vi "Periodic Tasks.vi"(8 "error in":errorcluster) -> ()   [LabVIEW 2013]
doc: "This VI runs in parallel to other tasks. It can contain as many user-defined periodic loops as you need. These can carry out PID or other sorts of timed response."
uses:
  <vilib>/Rock Robotics/SystemInterfaces/Typedef/FPGA_TypedefAnalogModule.ctl
  <vilib>/Rock Robotics/SystemInterfaces/Utilities/FPGA_UtilitiesLED Source.ctl
  <vilib>/Rock Robotics/SystemInterfaces/Utilities/FPGA_UtilitiesLED State.ctl
  <vilib>/Rock Robotics/WPI/Compressor/WPI_CompressorGetSetRefNum.vi
  Robot Global Data.vi
  <vilib>/Rock Robotics/WPI/RobotDrive/WPI_RobotDriveGetSetRefNum.vi
  <vilib>/Rock Robotics/WPI/Joystick/WPI_JoystickGetSetRefNum.vi
panel:
  out "distance":dbl(slide)=125.0 scale=0.0..250.0 scale format="%3d"
  in  "Scaling factor (V/in)":dbl=0.0098
  in  "Samples Per Second":dbl=1000.0
  in  "Average Bits":u8=3 max=15
  out "Encoder Rate (distance/sec)":dbl
  out "Encoder Distance":dbl
  out "Encoder Alarm Status":string
  out "Encoder Direction":string
  in  "Reset Encoder?":bool
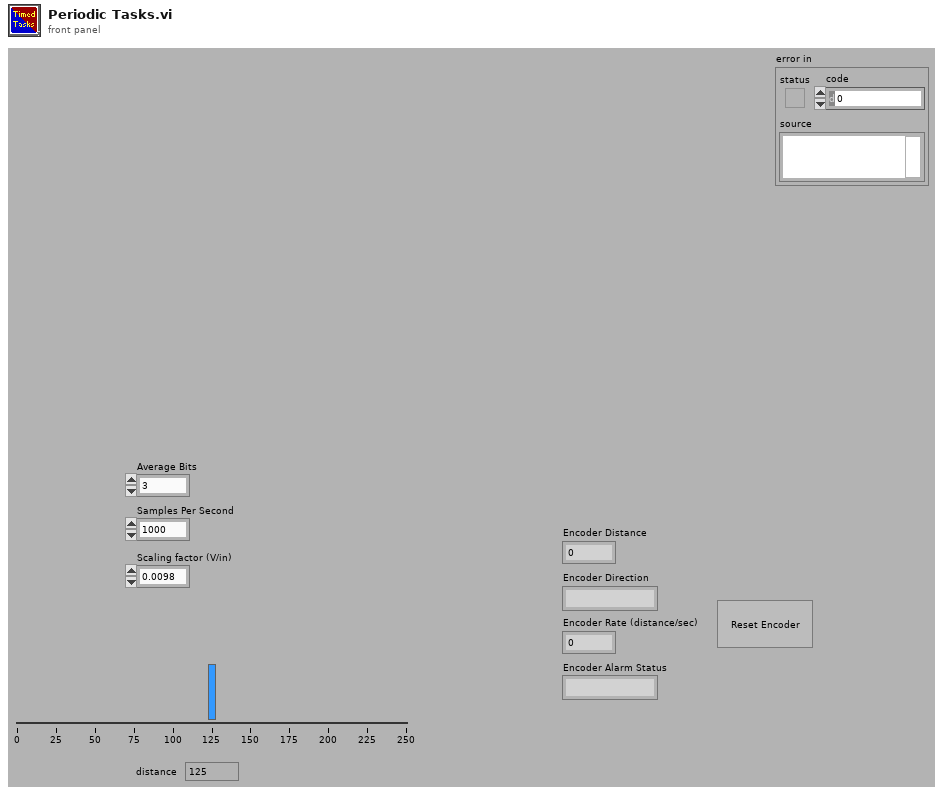
[diagram p1: front panel]
types:
  T1 = typedef "WPI_JoystickDevRef.ctl" = cluster{"Device":T2}
  T2 = typedef "WPI_JoystickDeviceEnum.ctl" = enum16{"USB 1", "USB 2", "USB 3", "USB 4", "Kinect 1", "Kinect 2"}
  T3 = typedef "WPI_RobotDriveDevRef.ctl" = cluster{"DevStatus":errorcluster, "Motors[]":T4[], "Square Inputs":bool, "Max Output":dbl, "Isochronous":bool}
  T4 = typedef "WPI_MotorControlDeviceRef.ctl" = cluster{"DeviceStatus":errorcluster, "Type":enum16{"PWM", "CAN"}, "PWM":cluster{"Digital Module":T5, "PWM Channel":T6, "DeadBand":T7}, "CAN":cluster{"Device Number":u8, "Control Mode":T8, "Semaphore":T9, "Max Vout":dbl}, "Invert":bool, "TransformRef":T10, "InvTransformRef":T10}
  T5 = typedef "FPGA_TypedefDigitalModule.ctl" = enum16{"Digital Module 1", "Digital Module 2"}
  T6 = typedef "FPGA_DIOPWMChannel.ctl" = enum8{"PWM 1", "PWM 2", "PWM 3", "PWM 4", "PWM 5", "PWM 6", "PWM 7", "PWM 8", "PWM 9", "PWM 10", "Invalid"}
  T7 = typedef "WPI_PWMDeadband.ctl" = cluster{"Name":string, "maxPositivePwm":i32, "minPositivePwm":i32, "centerPwm":i32, "maxNegativePwm":i32, "minNegativePwm":i32, "angularRange":u16}
  T8 = typedef "WPI_CANJaguar_ControlMode.ctl" = enum8{"Percent VBus", "Current", "Speed", "Position", "Voltage"}
  T9 = typedef "Semaphore RefNum" = refnum<k1>
  T10 = typedef "WPI_PWMTransform_ConPane.ctl" = refnum<vi>
  T11 = typedef "WPI_AnalogChannelDevRef.ctl" = cluster{"DevStatus":errorcluster, "Analog Module":T12, "Analog Channel":T13}
  T12 = typedef "FPGA_TypedefAnalogModule.ctl" = enum16{"Analog Module 1", "Analog Module 2"}
  T13 = typedef "FPGA_AIChannel.ctl" = enum8{"AI 1", "AI 2", "AI 3", "AI 4", "AI 5", "AI 6", "AI 7", "AI 8", "Invalid"}
  T14 = typedef "WPI_EncoderDevRef.ctl" = cluster{"DevStatus":errorcluster, "EncoderIndex":T15, "CounterIndex":T16, "DistancePerCount":dbl, "Decoding Type":T17}
  T15 = typedef "FPGA_EncoderIdx.ctl" = enum8{"Enc 0", "Enc 1", "Enc 2", "Enc 3", "Invalid"}
  T16 = typedef "FPGA_CounterCtrSystemIndex.ctl" = enum8{"Ctr 0", "Ctr 1", "Ctr 2", "Ctr 3", "Ctr 4", "Ctr 5", "Ctr 6", "Ctr 7", "Invalid"}
  T17 = typedef "WPI_EncoderType.ctl" = enum16{"1x", "2x", "4x"}
  T18 = cluster{"JoystickDevRef":T1, "RobotDriveDevRef":T3}
  T19 = typedef "FPGA_UtilitiesLED State.ctl" = enum16{"Off", "On", "Toggle"}
  T20 = typedef "FPGA_UtilitiesLED Source.ctl" = enum16{"User LED", "FPGA LED"}
  T21 = typedef "WPI_CompressorDevRef.ctl" = cluster{"DevStatus":errorcluster, "DigitalInputDevRef":T22, "RelayDevRef":T24}
  T22 = typedef "WPI_DigitalInputDevRef.ctl" = cluster{"DevStatus":errorcluster, "DIO Channel":T23, "Digital Module":T5}
  T23 = typedef "FPGA_DIOChannel.ctl" = enum8{"DIO 1", "DIO 2", "DIO 3", "DIO 4", "DIO 5", "DIO 6", "DIO 7", "DIO 8", "DIO 9", "DIO 10", "DIO 11", "DIO 12", "DIO 13", "DIO 14", "Invalid"}
  T24 = typedef "WPI_RelayDevRef.ctl" = cluster{"DevStatus":errorcluster, "Relay Channel":T25, "Digital Module":T5, "Relay Direction":T26}
  T25 = typedef "FPGA_DIORelayChannel.ctl" = enum8{"Relay 1", "Relay 2", "Relay 3", "Relay 4", "Relay 5", "Relay 6", "Relay 7", "Relay 8", "Invalid"}
  T26 = typedef "WPI_RelayDirection.ctl" = enum16{"Both directions", "Forward only", "Reverse only"}
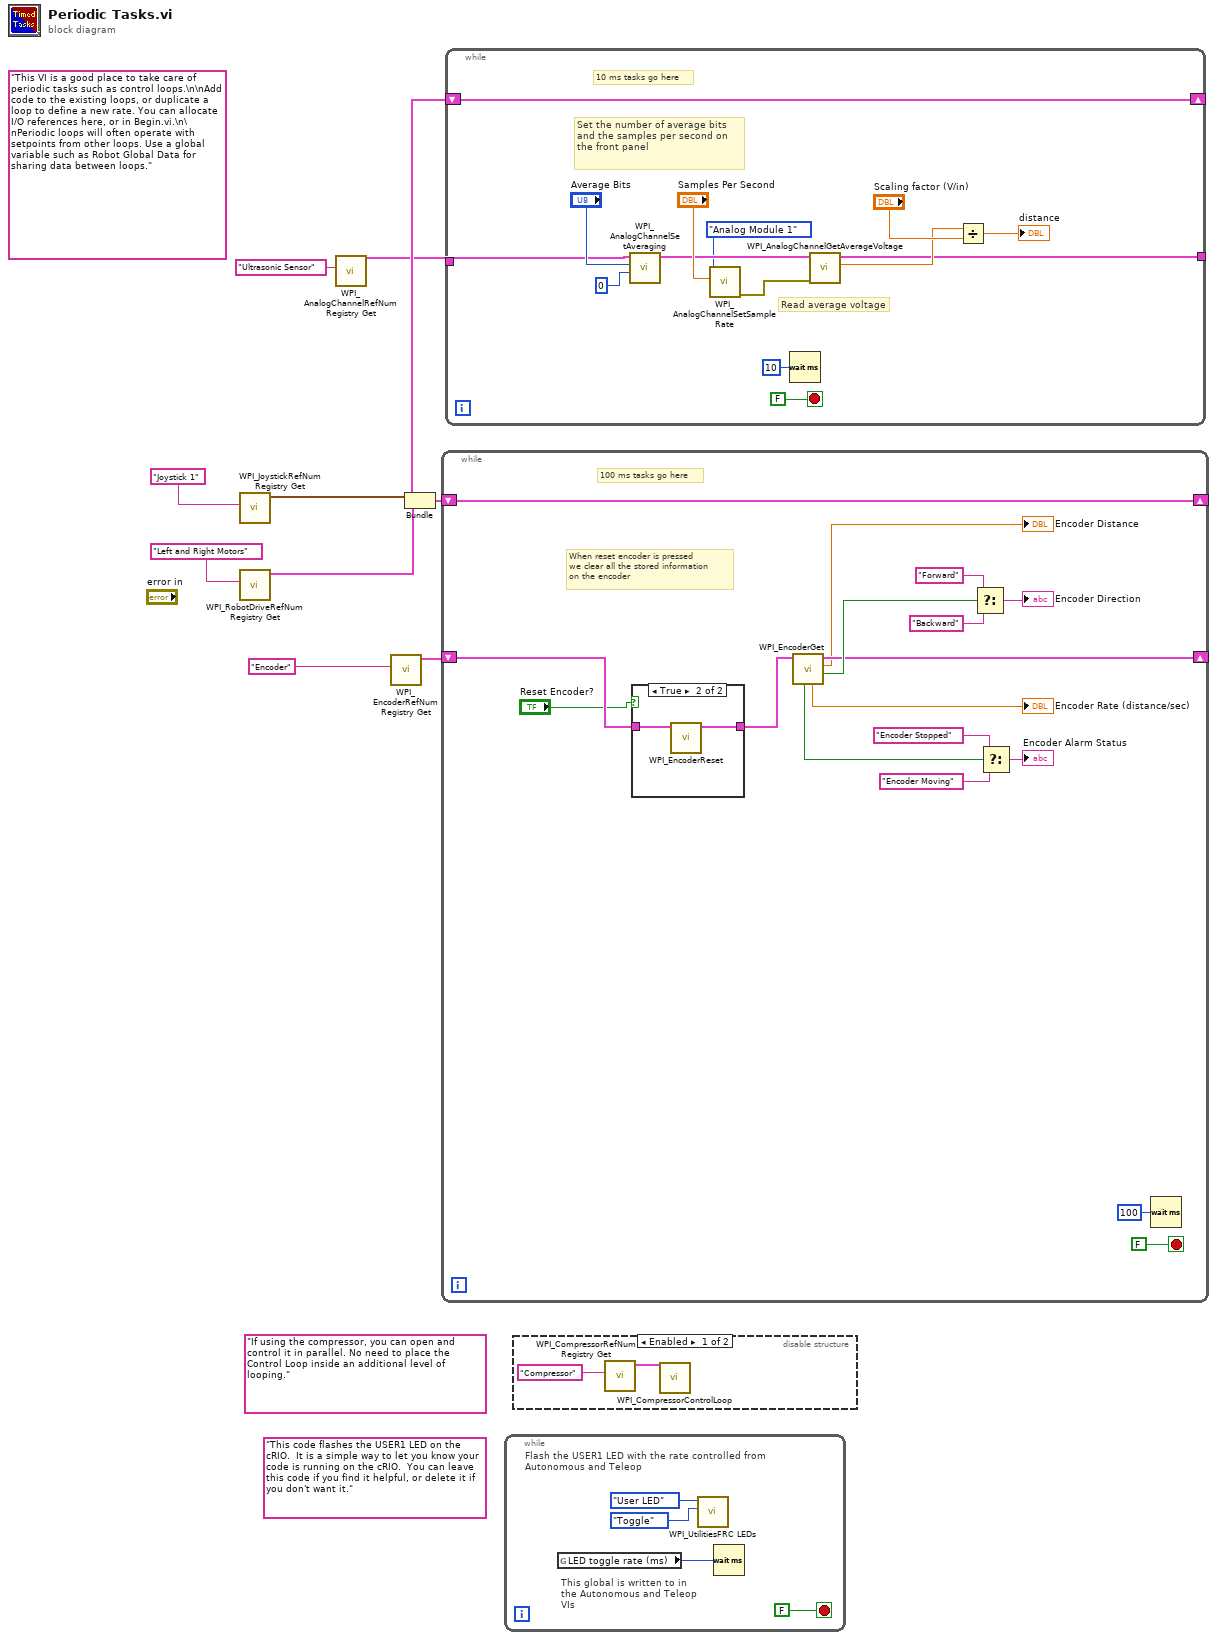
[diagram p0: block diagram]
diagram:
  (unwired) "If using the compressor, you can open and control it in parallel. No need to place the Control Loop inside an additional level of looping."
  (unwired) "This code flashes the USER1 LED on the cRIO.  It is a simple way to let you know your code is running on the cRIO.  You can leave this code if you find it helpful, or delete it if you don't want it."
  (unwired) "This VI is a good place to take care of periodic tasks such as control loops.\n\nAdd code to the existing loops, or duplicate a loop to define a new rate. You can allocate I/O references here, or in Begin.vi.\n\nPeriodic loops will often operate with setpoints from other loops. Use a global variable such as Robot Global Data for sharing data between loops."
  # "When reset encoder is pressed\nwe clear all the stored information\non the encoder"
  n1 = call <vilib>:"WPI_JoystickRefNum Registry Get.vi"("refnum name"="Joystick 1") -> ("JoystickDevRef"=w7:T1)  [unwired: 1 in, 9 out]
  n2 = call <vilib>:"WPI_RobotDriveRefNum Registry Get.vi"("refnum name"="Left and Right Motors") -> ("RobotDriveDevRef"=w6:T3)  [unwired: 1 in, 9 out]
  n3 = call <vilib>:"WPI_AnalogChannelRefNum Registry Get.vi"("refnum name"="Ultrasonic Sensor") -> ("AIDeviceRef"=w2:T11)  [unwired: 9 in, 1 out]
  n4 = call <vilib>:"WPI_EncoderRefNum Registry Get.vi"("refnum name"="Encoder") -> ("EncoderDevRef"=w4:T14)  [unwired: 9 in, 1 out]
  n5 = Bundle("JoystickDevRef"=w7, "RobotDriveDevRef"=w6) -> (w5:T18)  [unwired: 1 out]
  n6 = while {
    shift-right: [w24] -> _
    shift-left: w5 -> [w24]
    shift-right: [w12] -> _
    shift-left: w4 -> [w23]
    stop <- FALSE stop-if-true
    # "100 ms tasks go here"
    n7 = case shown="True" "Reset Encoder?" {
      tunnel: w23 -> [w27 w28]
      tunnel: [w27 w29] -> w13
      frame False {
      }
      frame True {
        n8 = call <vilib>:"WPI_EncoderReset.vi"("EncoderDevRef"=w28) -> ("EncoderDevRef"=w29:T14)  [unwired: 1 in, 9 out]
      }
    }
    n9 = call <vilib>:"WPI_EncoderGet.vi"("EncoderDevRef"=w13) -> ("Direction"=w16:bool, "Distance"=→"Encoder Distance":dbl, "EncoderDevRef"=w12:T14, "Rate"=→"Encoder Rate (distance/sec)":dbl, "Stopped"=w17:bool)  [unwired: 1 in, 5 out]
    n10 = Select(t="Forward", s=w16, f="Backward") -> (s? t:f=→"Encoder Direction":string)
    n11 = Select(t="Encoder Stopped", s=w17, f="Encoder Moving") -> (s? t:f=→"Encoder Alarm Status":string)
    n12 = Wait (ms)(milliseconds to wait=u32 100) -> ()  [unwired: 1 out]
  }
  n13 = while {
    shift-right: [w33] -> _
    shift-left: w5 -> [w33]
    tunnel: w2 -> [w32]
    tunnel: [w31] -> _
    stop <- FALSE stop-if-true
    # "Read average voltage"
    # "Set the number of average bits and the samples per second on the front panel"
    # "10 ms tasks go here"
    n14 = call <vilib>:"WPI_AnalogChannelSetAveraging.vi"("OversampleBits"=u8 0, "AverageBits"="Average Bits", "AIDeviceRef"=w32) -> ("AIDeviceRef"=w35:T11)  [unwired: 1 in, 7 out]
    n15 = call <vilib>:"WPI_AnalogChannelSetSampleRate.vi"("Samples Per Second"="Samples Per Second", "Analog Module (Module 1)"=FPGA_TypedefAnalogModule."Analog Module 1") -> ("error out"=w34:errorcluster)  [unwired: 2 in, 7 out]
    n16 = Wait (ms)(milliseconds to wait=u32 10) -> ()  [unwired: 1 out]
    n17 = call <vilib>:"WPI_AnalogChannelGetAverageVoltage.vi"("error in (no error)"=w34, "AIDeviceRef"=w35) -> ("Voltage"=w37:dbl, "AIDeviceRef"=w31:T11)  [unwired: 8 out]
    n18 = Divide(x=w37, y="Scaling factor (V/in)") -> (x/y=→"distance":dbl)
  }
  n19 = while {
    stop <- FALSE stop-if-true
    # "This global is written to in the Autonomous and Teleop VIs"
    # "Flash the USER1 LED with the rate controlled from Autonomous and Teleop"
    n20 = global read "Robot Global Data.vi" "LED toggle rate (ms)"() -> (w44:u32)
    n21 = call <vilib>:"WPI_UtilitiesFRC LEDs.vi"("State"=FPGA_UtilitiesLED_State."Toggle", "LED Type"=FPGA_UtilitiesLED_Source."User LED") -> ()  [unwired: 1 in, 9 out]
    n22 = Wait (ms)(milliseconds to wait=w44) -> ()  [unwired: 1 out]
  }
  n23 = disable-structure shown="Enabled" {
    frame Enabled {
      n24 = call <vilib>:"WPI_CompressorRefNum Registry Get.vi"("refnum name"="Compressor") -> ("CompressorDevRef"=w49:T21)  [unwired: 9 in, 1 out]
      n25 = call <vilib>:"WPI_CompressorControlLoop.vi"("CompressorDevRef"=w49) -> ()  [unwired: 11 in]
    }
    frame Disabled {
    }
  }
